vi "PurgePH3_01.vi"() -> ()   [LabVIEW 2011]
uses:
  <vilib>/Platform/TimedLoop/XDataNode/timing_clust.ctl
  <vilib>/Platform/TimedLoop/XDataNode/nitl_modes.ctl
  <vilib>/Platform/TimedLoop/XDataNode/wakeup.ctl
  <vilib>/Platform/TimedLoop/XDataNode/XDataNode.xnode
  <vilib>/Platform/TimedLoop/XDataNode/XDNodeRunTimeDep.lvlib
panel:
  in  "stop":bool
  in  "Numeric 3":dbl=30.0 caption="fill wait (s)"
  in  "Numeric 2":dbl=30.0 caption="evacuation wait (s)"
  out "As Gas Actual Flow Rate 2":dbl caption="evacuation flow"
  out "As Gas Actual Flow Rate":dbl caption="fill flow"
  out "Numeric":i32 caption="iteration"
  in  "y2":dbl=9.5 caption="fill threshold"
  in  "y":dbl=0.5 caption="evacuation threshold"
  in  "Iterations":i32=20
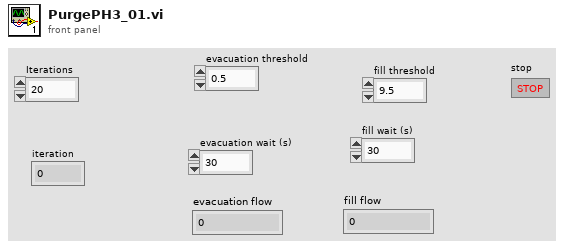
[diagram p1: front panel]
types:
  T1 = typedef "XDNodeRunTimeDep.lvlib/timing_clust.ctl" = cluster{"Expected End [f-1]":u64, "Actual End [f-1]":u64, "Finished Late? [f-1]":bool, "Expected End [i-1]":u64, "Actual End [i-1]":u64, "Finished Late? [i-1]":bool, "Expected Start [i]":u64, "Actual Start [i]":u64, "Expected Start [f]":u64, "Actual Start [f]":u64, "Source Name":string, "Structure Name":string, "Period":i64, "Deadline":i64, "Offset":i64, "Start":i64, "Priority":i32, "Timeout":i32, "Mode":T2, "Wakeup Reason":T3, "Error":errorcluster, "Source Type":string, "Secondary Source Type":string, "Global End Time":u64, "Global Start Time":u64, "Frame Duration":u64, "Iteration Duration":u64, "Assigned CPU":i32, "I/O Scan Engine Mode":u32}
  T2 = typedef "XDNodeRunTimeDep.lvlib/nitl_modes.ctl" = enum32{"No Change", "Process missed periods, maintain original phase", "Discard missed periods, maintain original phase", "Process missed periods, ignore original phase", "Discard missed periods, ignore original phase"}
  T3 = typedef "XDNodeRunTimeDep.lvlib/wakeup.ctl" = enum32{"Normal", "Aborted", "Asynchronous wakeup", "Timing source error", "Timed loop error", "Timeout"}
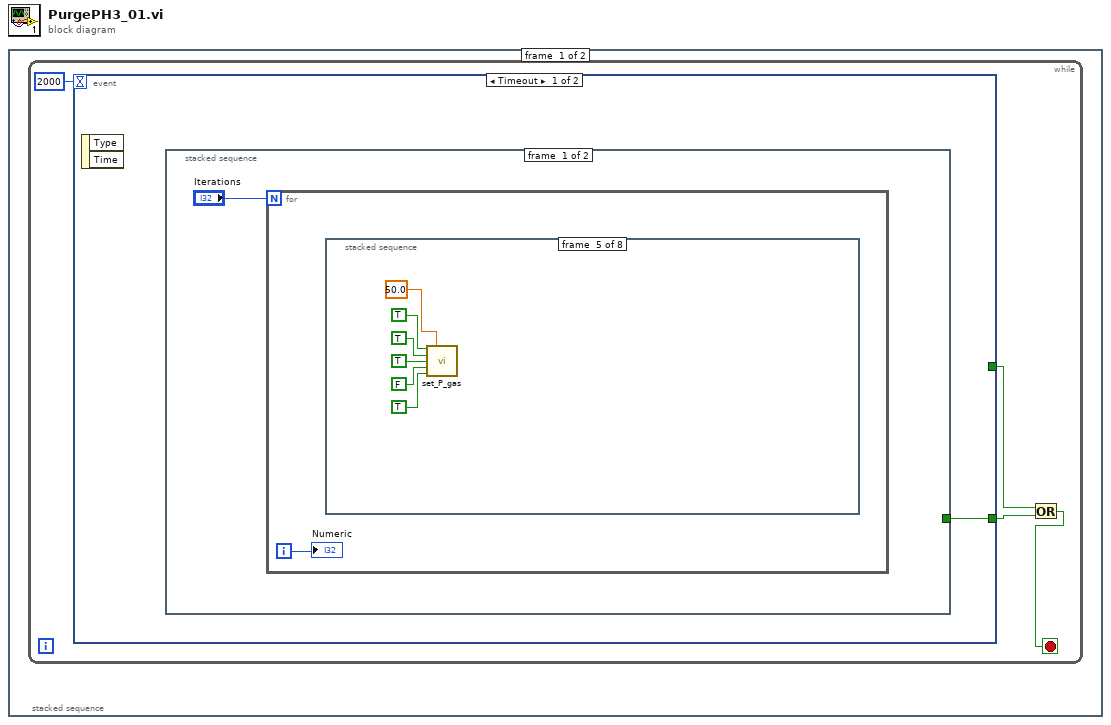
[diagram p0: block diagram]
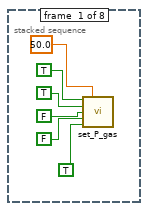
[diagram p2: hidden frame]
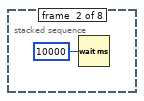
[diagram p3: hidden frame]
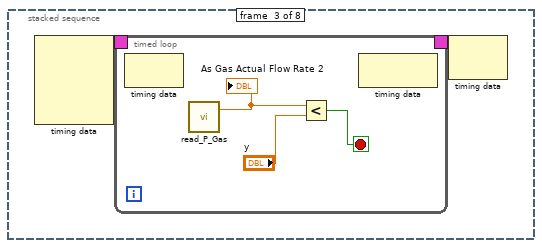
[diagram p4: hidden frame]
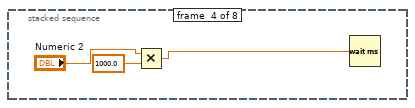
[diagram p5: hidden frame]
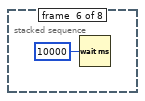
[diagram p6: hidden frame]
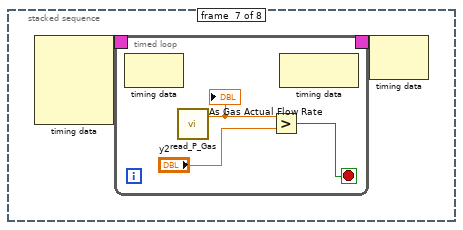
[diagram p7: hidden frame]
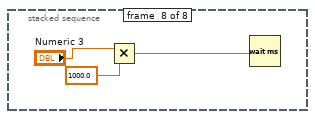
[diagram p8: hidden frame]
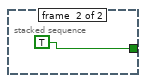
[diagram p9: hidden frame]
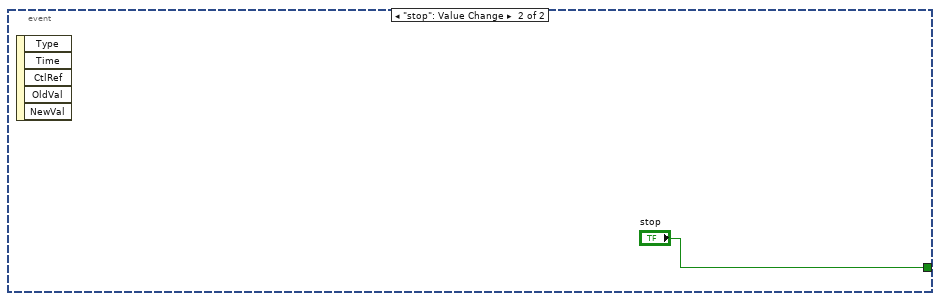
[diagram p10: hidden frame]
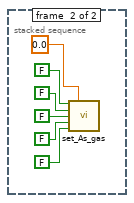
[diagram p11: hidden frame]
diagram:
  n1 = stacked-sequence {
    frame #0 {
      n2 = while {
        stop <- w2 stop-if-true
        n3 = event shown="[0] Timeout" {
          selector: _ -> [_ _]
          dyn-events: _ -> [_ _]
          timeout: 2000 -> [_ _]
          tunnel: [_ "stop"] -> w3
          tunnel: [w5 _] -> w4
          event Timeout {
            n4 = event-data() -> ()  [unwired: 1 in, 2 out]
            n5 = stacked-sequence {
              tunnel: [_ TRUE] -> w5
              frame #0 {
                n6 = for {
                  N: "Iterations" -> [_]
                  i -> [w7]
                  n7 = stacked-sequence {
                    frame #0 {
                      n8 = call "set_P_gas.vi"("P_Gas Active"=TRUE ("As_Gas Active"), "P_Gas Flow"=50.0 ("As_Gas Flow"), "P_Gas In"=TRUE ("As_Gas In"), "P_Gas H2 In"=FALSE ("As_Gas H2"), "P_Gas Run"=FALSE ("As_Gas Run"), "P_Gas Remote"=TRUE ("As_Gas Remote")) -> ()  [unwired: 10 in]
                    }
                    frame #1 {
                      n9 = Wait (ms)(milliseconds to wait=u32 10000) -> ()  [unwired: 1 out]
                    }
                    frame #2 {
                      n10 = node-c288() -> (w16:T1)  [unwired: 4 in]
                      n11 = timed-loop {
                        timing: w16 -> [_]
                        timing-out: [_] -> w15
                        stop <- w17 stop-if-true
                        n12 = node-c288() -> ()  [unwired: 1 in, 1 out]
                        n13 = call "read_P_Gas.vi"() -> ("P Gas Actual Flow Rate"=w19:dbl)  [unwired: 5 out]
                        "As Gas Actual Flow Rate 2" <- w19
                        n14 = Less?(x=w19, y="y") -> (x < y?=w17:bool)
                        n15 = node-c288() -> ()  [unwired: 1 in, 1 out]
                      }
                      n16 = node-c288(w15) -> ()  [unwired: 1 out]
                    }
                    frame #3 {
                      n17 = Multiply(x="Numeric 2", y=1000.0) -> (x*y=w24:dbl)
                      n18 = Wait (ms)(milliseconds to wait=w24) -> ()  [unwired: 1 out]
                    }
                    frame #4 {
                      n19 = call "set_P_gas.vi"("P_Gas Active"=TRUE ("As_Gas Active"), "P_Gas Flow"=50.0 ("As_Gas Flow"), "P_Gas In"=TRUE ("As_Gas In"), "P_Gas H2 In"=TRUE ("As_Gas H2"), "P_Gas Run"=FALSE ("As_Gas Run"), "P_Gas Remote"=TRUE ("As_Gas Remote")) -> ()  [unwired: 10 in]
                    }
                    frame #5 {
                      n20 = Wait (ms)(milliseconds to wait=u32 10000) -> ()  [unwired: 1 out]
                    }
                    frame #6 {
                      n21 = node-c288() -> (w35:T1)  [unwired: 4 in]
                      n22 = timed-loop {
                        timing: w35 -> [_]
                        timing-out: [_] -> w34
                        stop <- w36 stop-if-true
                        n23 = node-c288() -> ()  [unwired: 1 in, 1 out]
                        n24 = call "read_P_Gas.vi"() -> ("P Gas Actual Flow Rate"=w38:dbl)  [unwired: 5 out]
                        "As Gas Actual Flow Rate" <- w38
                        n25 = Greater?(x=w38, y="y2") -> (0:w36:bool)
                        n26 = node-c288() -> ()  [unwired: 1 in, 1 out]
                      }
                      n27 = node-c288(w34) -> ()  [unwired: 1 out]
                    }
                    frame #7 {
                      n28 = Multiply(x="Numeric 3", y=1000.0) -> (x*y=w43:dbl)
                      n29 = Wait (ms)(milliseconds to wait=w43) -> ()  [unwired: 1 out]
                    }
                  }
                  "Numeric" <- w7
                }
              }
              frame #1 {
              }
            }
          }
          event "stop": Value Change {
            n30 = event-data() -> ()  [unwired: 1 in, 5 out]
          }
        }
        n31 = Or(x=w3, y=w4) -> (x .or. y?=w2:bool)
      }
    }
    frame #1 {
      n32 = call "set_As_gas.vi"("As_Gas Active"=FALSE, "As_Gas Flow"=0.0, "As_Gas In"=FALSE, "As_Gas H2"=FALSE, "As_Gas Run"=FALSE, "As_Gas Remote"=FALSE) -> ()  [unwired: 10 in]
    }
  }
